vi "DownsampleWaveform.vi"(9 "dt":dbl, 10 "Number of Samples":i32, 11 "data":sgl[](array[numeric])) -> (1 "new dt":dbl, 3 "values":sgl[](array[numeric]))   [LabVIEW 2017, in "CmsTestPanel.lvlib"]
uses:
  <vilib>/addons/InsightCM/Devices/Shared/Cms/CmsTestPanel/CmsTestPanel.lvlib
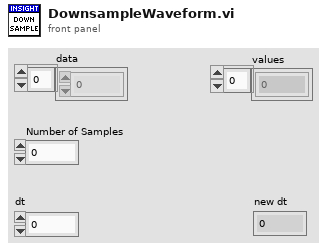
[diagram p1: front panel]
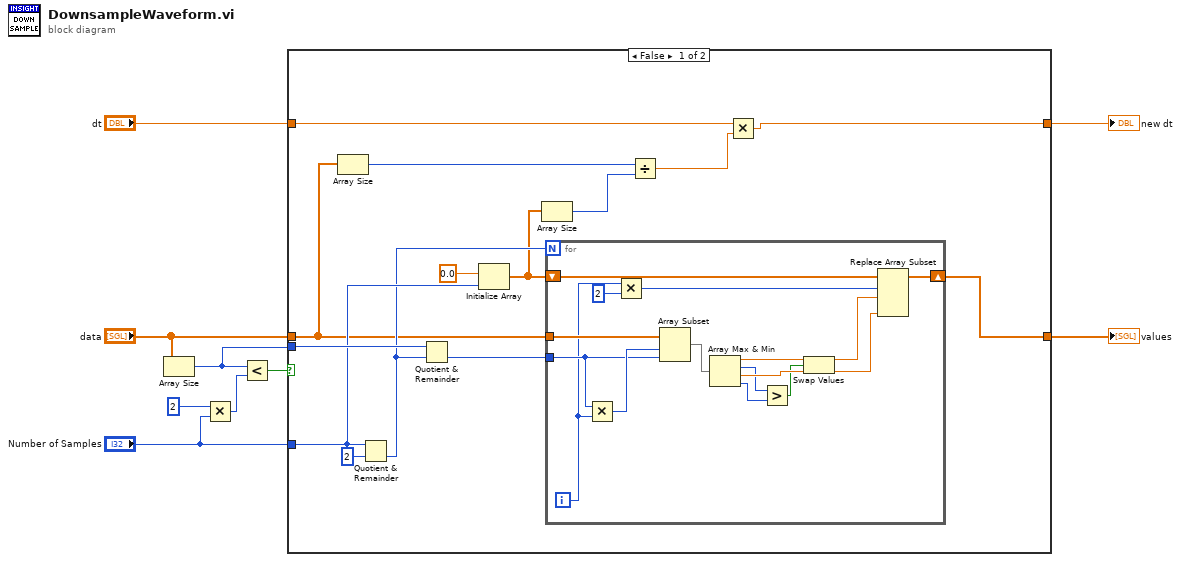
[diagram p0: block diagram]
diagram:
  n1 = Array Size(array="data") -> (size(s)=w3:i32)
  n2 = Multiply(x=2, y="Number of Samples") -> (x*y=w9:i32)
  n3 = Less?(x=w3, y=w9) -> (x < y?=w7:bool)
  n4 = case shown="False" w7 {
    tunnel: [w19 w41] -> w6
    tunnel: "data" -> [w16 w41]
    tunnel: "Number of Samples" -> [w18 _]
    tunnel: w3 -> [w22 _]
    tunnel: "dt" -> [w12 w40]
    tunnel: [w10 w40] -> w1
    frame False {
      n5 = Array Size(array=w16) -> (size(s)=w14:i32)
      n6 = Quotient & Remainder(x=w18, y=2) -> (floor(x/y)=w17:i32)  [unwired: 1 out]
      n7 = Quotient & Remainder(x=w22, y=w17) -> (floor(x/y)=w21:i32)  [unwired: 1 out]
      n8 = Initialize Array(sgl 0.0, w18) -> (w15:sgl[])
      n9 = Array Size(array=w15) -> (size(s)=w13:i32)
      n10 = for {
        N: w17 -> [_]
        tunnel: w16 -> [w39]
        tunnel: w21 -> [w37]
        shift-right: [w34] -> w19
        shift-left: w15 -> [w35]
        i -> [w25]
        n11 = Multiply(x=w37, y=w25) -> (x*y=w38:i32)
        n12 = Multiply(x=w25, y=2) -> (x*y=w24:i32)
        n13 = Array Subset(array=w39, index=w38, length=w37) -> (w36:sgl[])
        n14 = Array Max & Min(array=w36) -> (max value=w33:sgl, max index (indices)=w31:i32, min value=w32:sgl, min index (indices)=w30:i32)
        n15 = Greater?(x=w31, y=w30) -> (0:w29:bool)
        n16 = Swap Values(12:w33, 13:w29, 14:w32) -> (1:w28:sgl, 3:w27:sgl)
        n17 = Replace Array Subset(array=w35, new element #1=w28, index #1=w24, new element #2=w27) -> (w34:sgl[])  [unwired: 1 in]
      }
      n18 = Divide(x=w14, y=w13) -> (x/y=w11:dbl)
      n19 = Multiply(x=w12, y=w11) -> (x*y=w10:dbl)
    }
    frame True {
    }
  }
  "values" <- w6
  "new dt" <- w1
